vi "test_si.vi"() -> ()   [LabVIEW 2023]
panel:
  out "right_hand":T1(array[cluster])
  out "left_hand":T1(array[cluster])
  out "eye_ray":sgl[](array[numeric])
  out "head_pose":sgl[](array[numeric])
  out "valid":u32
  in  "stop":bool
  in  "host":string="192.168.1.7"
  in  "path in":path=path "C:/Users/jcds/Documents/GitHub/hl2ss/extensions/client_labview/hl2ss_labview/hl2ss_ulm.dll"
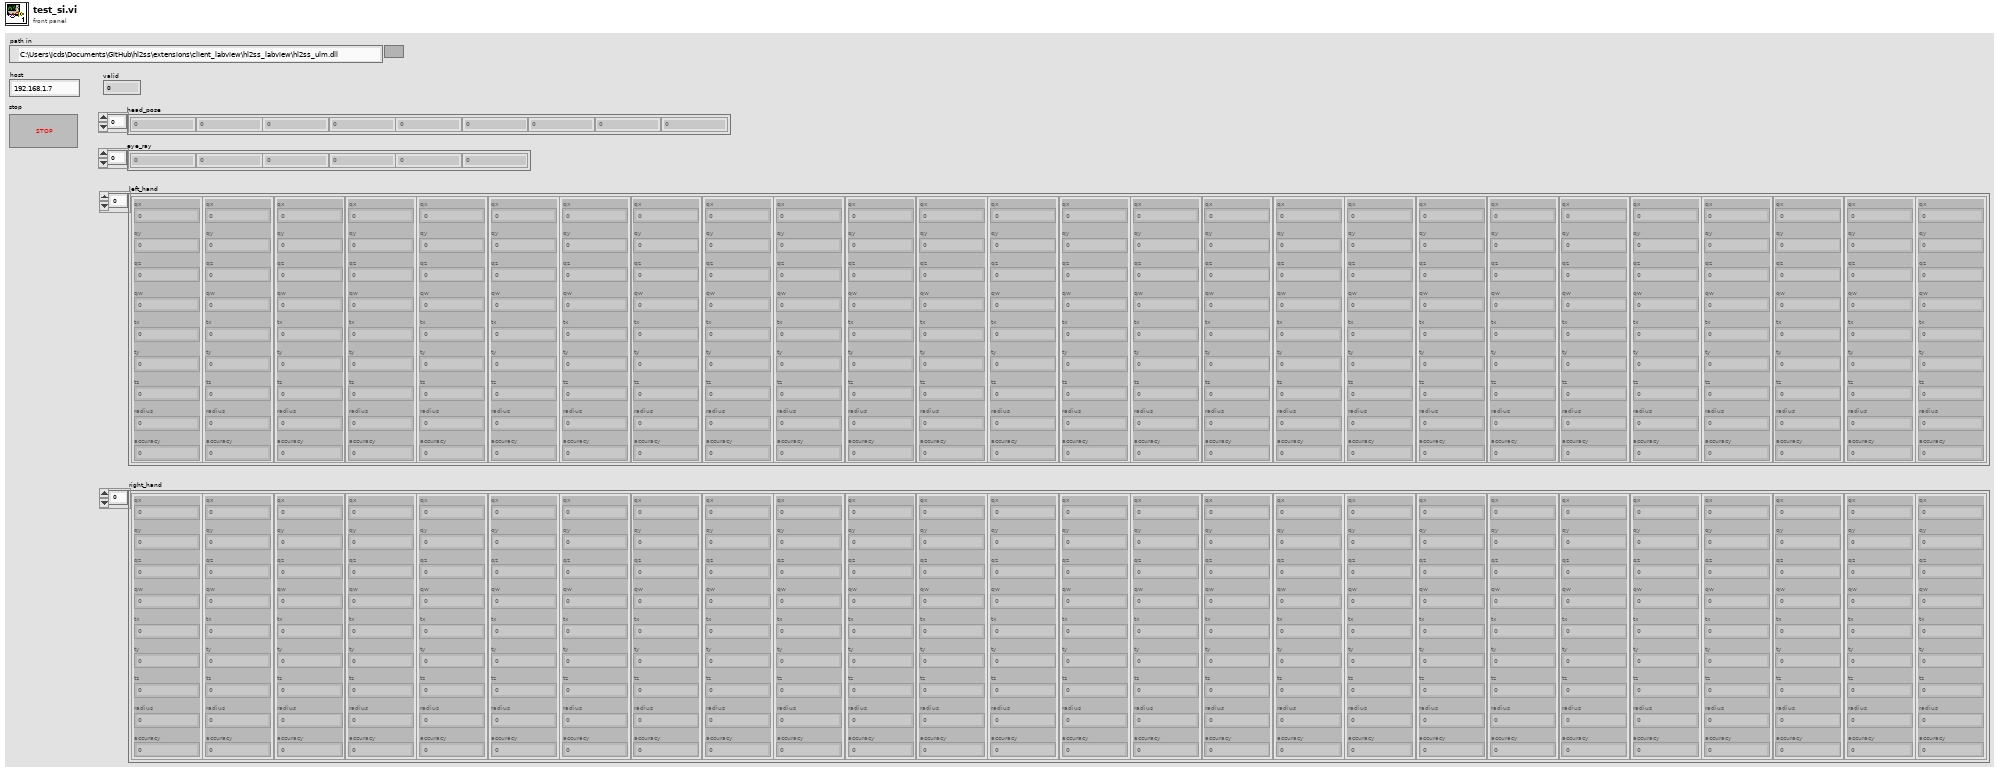
[diagram p1: front panel]
types:
  T1 = cluster{"qx":sgl, "qy":sgl, "qz":sgl, "qw":sgl, "tx":sgl, "ty":sgl, "tz":sgl, "radius":sgl, "accuracy":i32}[]
  T2 = cluster{"frame_stamp":i64, "timestamp":u64, "payload_size":u32, "status":i32, "payload":u64, "pose":u64}
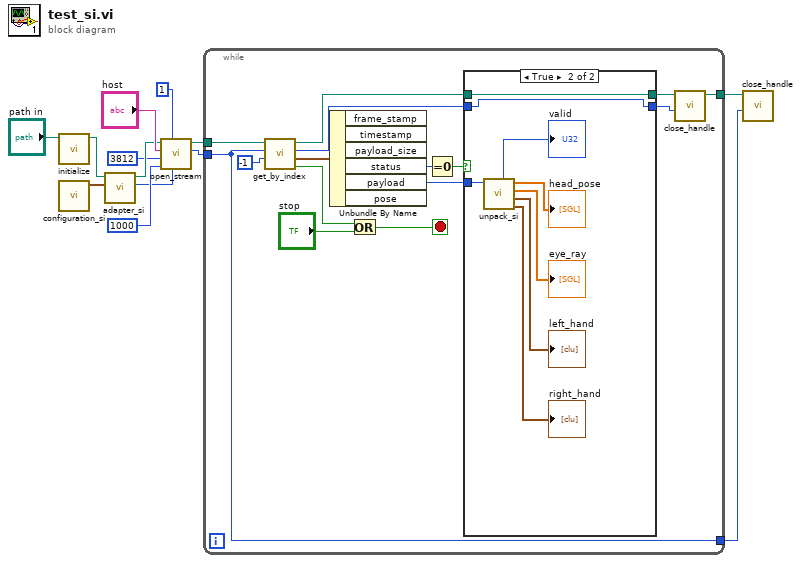
[diagram p0: block diagram]
diagram:
  n1 = call "initialize.vi"("path in"="path in") -> ("path out"=w4:path)  [unwired: 9 in, 1 out]
  n2 = call "configuration_si.vi"() -> ("configuration_si"=w2:cluster{"chunk":u64})  [unwired: 11 in]
  n3 = call "adapter_si.vi"("configuration_si"=w2, "path in"=w4) -> ("configuration"=w6:u64, "path out"=w5:path)  [unwired: 8 in]
  n4 = call "open_stream.vi"("configuration"=w6, "decoded"=u8 1, "buffer_size"=u64 1000, "port"=u16 3812, "host"="host", "path in"=w5) -> ("handle"=w9:u64, "path out"=w10:path)  [unwired: 3 in, 1 out]
  n5 = while {
    tunnel: w10 -> [w28]
    tunnel: w9 -> [w14]
    tunnel: [w15] -> w8
    tunnel: [w14] -> w7
    stop <- w26 stop-if-true
    n6 = call "get_by_index.vi"("frame_stamp"=i64 -1, "stream_handle"=w14, "path in"=w28) -> ("error"=w25:bool, "packet"=w23:T2, "packet_handle"=w18:u64, "path out"=w19:path)  [unwired: 5 in]
    n7 = Unbundle By Name(w23) -> ("status"=w21:i32, "payload"=w22:u64)  [unwired: 4 out]
    n8 = Or(x=w25, y="stop") -> (x .or. y?=w26:bool)
    n9 = Equal To 0?(x=w21) -> (x = 0?=w20:bool)
    n10 = case shown="True" w20 {
      tunnel: w22 -> [_ w36]
      tunnel: w19 -> [w29 w38]
      tunnel: w18 -> [w30 w37]
      tunnel: [w29 w38] -> w17
      tunnel: [w30 w37] -> w16
      frame False {
      }
      frame True {
        n11 = call "unpack_si.vi"("payload"=w36) -> ("right_hand"=→"right_hand":T1, "left_hand"=→"left_hand":T1, "eye_ray"=→"eye_ray":sgl[], "head_pose"=→"head_pose":sgl[], "valid"=→"valid":u32)  [unwired: 5 in, 1 out]
      }
    }
    n12 = call "close_handle.vi"("handle"=w16, "path in"=w17) -> ("path out"=w15:path)  [unwired: 9 in]
  }
  n13 = call "close_handle.vi"("handle"=w7, "path in"=w8) -> ()  [unwired: 9 in, 1 out]
